vi "Initiate.vi"(0 "device session in":refnum<class "Device Session.lvclass">, 11 "error in":errorcluster) -> (4 "device session out":refnum<class "Device Session.lvclass">, 15 "error out":errorcluster)   [LabVIEW 2015, in "Device Session.lvclass"]
doc: "Initiates a new acquisition from the FPGA. You must configure the acquisition by running the <B>Configure Acquisition</B> VI before running this VI.\n\n<B>Input Parameters</B>\n\n<B>device session in</B> is a reference to the session containing sessions to all instrument design libraries used in this sample project. This parameter is obtained from the 'Open Session' VI.\n\n<B>error in</B> describes error conditions that occur before this node runs. This input provides standard 'error in' functionality.\n\n<B>Output Parameters</B>\n\n<B>device session out</B> passes a reference to the session to the next VI.\n\n<B>error out</B> contains error information. This output provides standard 'error out' functionality."
uses:
  Device Session.lvclass
  Device Session.lvclass/Device Session.ctl
  FPGA Refnum.ctl
  <vilib>/Utility/error.llb/Error Cluster From Error Code.vi
  <vilib>/rvi/errors/niLvFpgaAdjustHostInterfaceError.vi
  <vilib>/rvi/interface/nirviReadWriteControl/nirviReadWriteControl.xnode
  <vilib>/rvi/interface/nirviMethod/nirviMethod.xnode
  <instrlib>/HSAI-RIO/Config/Interface/v1/Host/niHSAI Config v1 Host.lvclass
  <vilib>/rvi/errors/niLvFpgaMergeErrorWithErrorCode.vi
  NiFpgaLv.dll
  <vilib>/rvi/interface/Simulation/niFpgaSimulationCallBeginRW.vi
  <vilib>/FPGAPlugInAG/Dynamic/niLvFpga_ReadFifo_Dynamic.vi
  <vilib>/FPGAPlugInAG/Dynamic/niLvFpga_StopFifo_Dynamic.vi
  <vilib>/FPGAPlugInAG/Dynamic/niLvFpga_StartFifo_Dynamic.vi
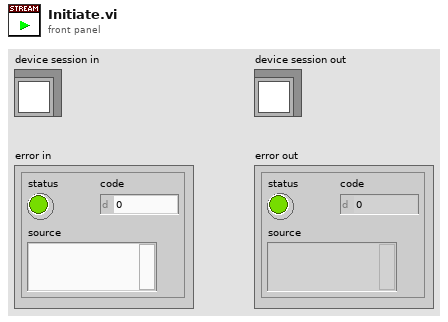
[diagram p1: front panel]
types:
  T1 = typedef "Device Session.lvclass/FPGA Refnum.ctl" = refnum<k20>
  T2 = typedef "Device Session.lvclass/Device Session Object.ctl" = cluster{"ni5171R FPGA Reference":T1, "niHSAI config":refnum<class "niHSAI Config v1 Host.lvclass">, "configured scaling coefficients":cluster{"gain":dbl, "offset":dbl}[], "number of channels to stream":u8, "selected acq channels":bool[], "number of channels":u32, "actual channel configuration":T3[], "configured channels":bool[], "sample clock rate (Hz)":dbl}
  T3 = typedef "niHSAI Types v1 Host.lvlib/Channel Configuration.ctl" = cluster{"channel":u32, "coupling":T4, "impedance":T5, "bandwidth":T6, "vertical range":dbl, "vertical offset":dbl}
  T4 = typedef "niHSAI Types v1 Host.lvlib/Coupling.ctl" = enum8{"Default", "DC", "AC"}
  T5 = typedef "niHSAI Types v1 Host.lvlib/Impedance.ctl" = enum8{"Default", "1 mega ohm", "50 ohm"}
  T6 = typedef "niHSAI Types v1 Host.lvlib/Bandwidth.ctl" = enum8{"Default", "Full Bandwidth", "Anti-alias Filter"}
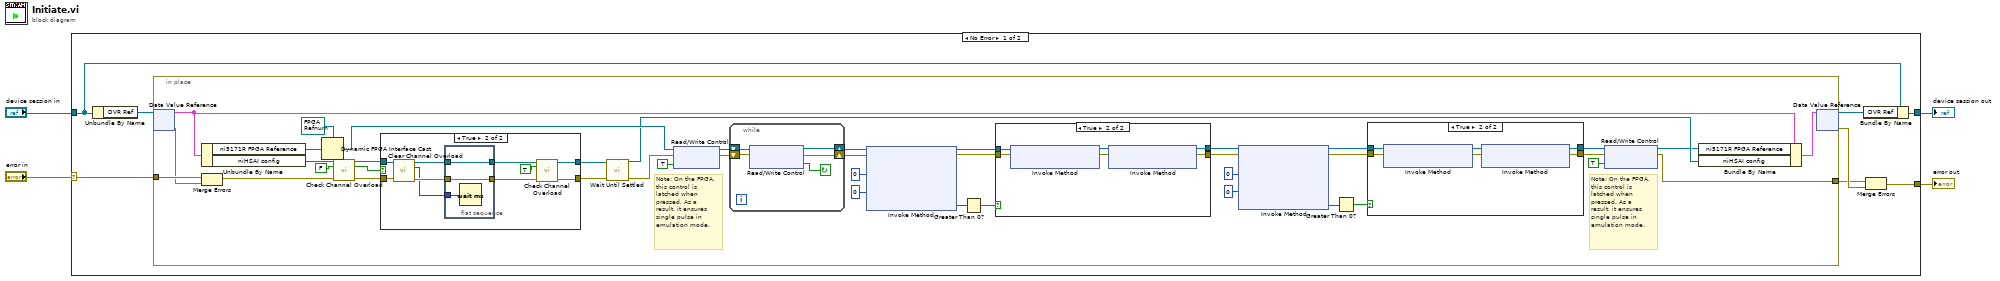
[diagram p0: block diagram]
diagram:
  n1 = case shown="No Error" "error in" {
    selector: "error in" -> [w6 w91]
    tunnel: "device session in" -> [w11 w90]
    tunnel: [w8 w91] -> w3
    tunnel: [w9 w90] -> w2
    frame No Error {
      n2 = Unbundle By Name(w11) -> ("DVR Ref"=w12:refnum<data-value>)
      n3 = in-place {
        in-place-border: w6 -> [w51]
        in-place-border: [w31] -> w5
        # "Note: On the FPGA, this control is latched when pressed. As a result, it ensures single pulse in emulation mode."
        # "Note: On the FPGA, this control is latched when pressed. As a result, it ensures single pulse in emulation mode."
        n4 = in-place-dvr #1(w12) -> (w52:T2, w50:errorcluster)
        n5 = Merge Errors(w51, w50) -> (w18:errorcluster)
        n6 = Unbundle By Name(w52) -> ("ni5171R FPGA Reference"=w47:T1, "niHSAI config"=w20:refnum<class "niHSAI Config v1 Host.lvclass">)
        n7 = Dynamic FPGA Interface Cast(Session In=T1 refnum ("FPGA Interface"), Type=w47) -> (Session Out=w46:T1)
        n8 = call-dynamic "Check Channel Overload.vi"("session in"=w20, "set error? (T)"=FALSE, "error in"=w18) -> ("session out"=w14:refnum<class "niHSAI Config v1 Host.lvclass">, "overloaded?"=w17:bool, "error out"=w15:errorcluster)  [unwired: 10 in]
        n9 = case shown="True" w17 {
          tunnel: [w54 w57] -> w16
          tunnel: w15 -> [w54 w65]
          tunnel: w14 -> [w55 w64]
          tunnel: [w55 w56] -> w13
          frame False {
          }
          frame True {
            n10 = call-dynamic "Clear Channel Overload.vi"("session in"=w64, "error in"=w65) -> ("session out"=w62:refnum<class "niHSAI Config v1 Host.lvclass">, "min wait time (ms)"=w61:u32, "error out"=w63:errorcluster)  [unwired: 11 in]
            n11 = flat-sequence {
              tunnel: w63 -> [w67]
              tunnel: w62 -> [w66]
              tunnel: w61 -> [w68]
              tunnel: [w67] -> w60
              tunnel: [w66] -> w59
              frame #0 {
                n12 = Wait (ms)(milliseconds to wait=w68) -> ()  [unwired: 1 out]
              }
            }
            n13 = call-dynamic "Check Channel Overload.vi"("session in"=w59, "set error? (T)"=TRUE, "error in"=w60) -> ("session out"=w56:refnum<class "niHSAI Config v1 Host.lvclass">, "error out"=w57:errorcluster)  [unwired: 10 in, 1 out]
          }
        }
        n14 = call-dynamic "Wait Until Settled.vi"("session in"=w13, "error in"=w16) -> ("session out"=w38:refnum<class "niHSAI Config v1 Host.lvclass">, "error out"=w39:errorcluster)  [unwired: 12 in]
        n15 = xnode "Read/Write Control"("FPGA VI Reference In"=w46, "error in"=w39, "acq.reset"=TRUE ("acq.enabled")) -> ("FPGA VI Reference Out"=w37:T1, "error out"=w36:errorcluster)
        n16 = while {
          shift-right: [w79] -> w35
          shift-left: w37 -> [w81]
          shift-right: [w78] -> w34
          shift-left: w36 -> [w80]
          stop <- w77 continue-if-true
          n17 = xnode "Read/Write Control"("FPGA VI Reference In"=w81, "error in"=w80) -> ("FPGA VI Reference Out"=w79:T1, "error out"=w78:errorcluster, "acq.in reset"=w77:bool)
        }
        n18 = xnode "Invoke Method"("FPGA VI Reference In"=w35, "error in"=w34, "Number of Elements"=u32 0, "Timeout (ms)"=0) -> ("FPGA VI Reference Out"=w42:T1, "error out"=w41:errorcluster, "Elements Remaining"=w43:u32)  [unwired: 1 out]
        n19 = Greater Than 0?(x=w43) -> (x > 0?=w40:bool)
        n20 = case shown="True" w40 {
          tunnel: w42 -> [w83 w89]
          tunnel: w41 -> [w82 w88]
          tunnel: [w83 w85] -> w23
          tunnel: [w82 w84] -> w24
          frame False {
          }
          frame True {
            n21 = xnode "Invoke Method"("FPGA VI Reference In"=w89, "error in"=w88) -> ("FPGA VI Reference Out"=w87:T1, "error out"=w86:errorcluster)
            n22 = xnode "Invoke Method"("FPGA VI Reference In"=w87, "error in"=w86) -> ("FPGA VI Reference Out"=w85:T1, "error out"=w84:errorcluster)
          }
        }
        n23 = xnode "Invoke Method"("FPGA VI Reference In"=w23, "error in"=w24, "Number of Elements"=u32 0, "Timeout (ms)"=0) -> ("FPGA VI Reference Out"=w28:T1, "error out"=w29:errorcluster, "Elements Remaining"=w27:u32)  [unwired: 1 out]
        n24 = Greater Than 0?(x=w27) -> (x > 0?=w30:bool)
        n25 = case shown="True" w30 {
          tunnel: w28 -> [w70 w76]
          tunnel: w29 -> [w69 w75]
          tunnel: [w70 w72] -> w22
          tunnel: [w69 w71] -> w21
          frame False {
          }
          frame True {
            n26 = xnode "Invoke Method"("FPGA VI Reference In"=w76, "error in"=w75) -> ("FPGA VI Reference Out"=w74:T1, "error out"=w73:errorcluster)
            n27 = xnode "Invoke Method"("FPGA VI Reference In"=w74, "error in"=w73) -> ("FPGA VI Reference Out"=w72:T1, "error out"=w71:errorcluster)
          }
        }
        n28 = xnode "Read/Write Control"("FPGA VI Reference In"=w22, "error in"=w21, "acq.initiate"=TRUE ("acq.enabled")) -> ("FPGA VI Reference Out"=w32:T1, "error out"=w31:errorcluster)
        n29 = Bundle By Name(cluster=w52, "ni5171R FPGA Reference"=w32, "niHSAI config"=w38) -> (w49:T2)
        n30 = in-place-dvr #1(w49) -> (w10:refnum<data-value>, w7:errorcluster)
      }
      n31 = Bundle By Name(cluster=w11, "DVR Ref"=w10) -> (w9:refnum<class "Device Session.lvclass">)
      n32 = Merge Errors(w5, w7) -> (w8:errorcluster)
    }
    frame Error {
    }
  }
  "error out" <- w3
  "device session out" <- w2
